vi "LD2018_ブロック崩し_Command受取.vi"(0 "Start":bool, 1 "Combo":i32, 5 "Stage入力":i32, 7 "残機入力":i32, 9 "Play中入力":bool, 11 "Cue timed out":bool, 12 "Command":string) -> (3 "Combo出力":i32, 4 "Start出力":bool, 6 "Stage出力":i32, 8 "残機出力":i32, 10 "Play中出力":bool, 15 "Quit?":bool)   [LabVIEW 2017]
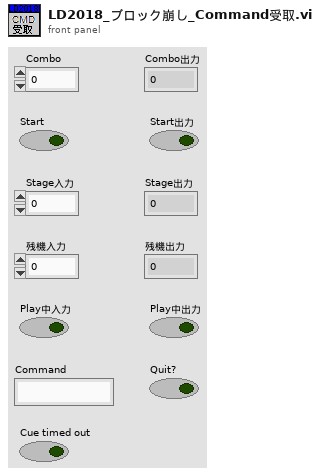
[diagram p1: front panel]
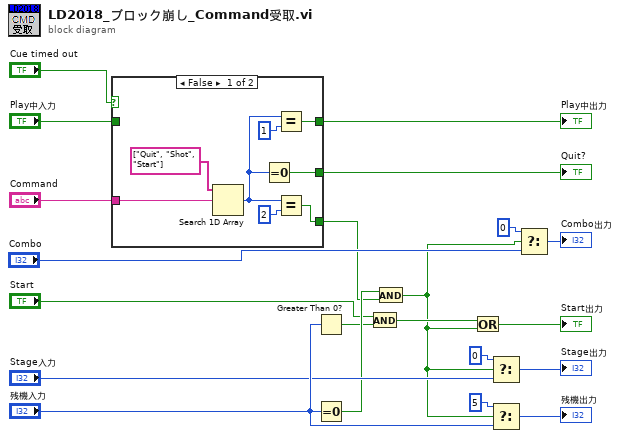
[diagram p0: block diagram]
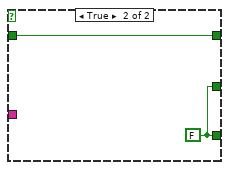
[diagram p2: hidden frame]
diagram:
  n1 = case shown="FALSE" "Cue timed out" {
    tunnel: "Command" -> [w28 _]
    tunnel: [w27 w30] -> w5
    tunnel: [w22 w31] -> w2
    tunnel: "Play中入力" -> [_ w31]
    tunnel: [w24 w30] -> w11
    frame False {
      n2 = Search 1D Array(1D array=string[] ["Quit", "Shot", "Start"], element=w28) -> (index of element=w26:i32)  [unwired: 1 in]
      n3 = Equal To 0?(x=w26) -> (x = 0?=w27:bool)
      n4 = Equal?(x=w26, y=1) -> (x = y?=w22:bool)
      n5 = Equal?(x=w26, y=2) -> (x = y?=w24:bool)
    }
    frame True {
      w30 = FALSE
    }
  }
  "Play中出力" <- w2
  "Quit?" <- w5
  n6 = Greater Than 0?(x="残機入力") -> (x > 0?=w10:bool)
  n7 = Equal To 0?(x="残機入力") -> (x = 0?=w12:bool)
  n8 = And(x="Start", y=w10) -> (x .and. y?=w8:bool)
  n9 = And(x=w12, y=w11) -> (x .and. y?=w1:bool)
  n10 = Or(x=w8, y=w1) -> (x .or. y?=→"Start出力":bool)
  n11 = Select(t=0, s=w1, f="Stage入力") -> (s? t:f=→"Stage出力":i32)
  n12 = Select(t=5, s=w1, f="残機入力") -> (s? t:f=→"残機出力":i32)
  n13 = Select(t=0, s=w1, f="Combo") -> (s? t:f=→"Combo出力":i32)
